vi "ramp.vi"(4 "DigNum Refnum":refnum<vi>, 5 "Bool Refnum Reset":refnum<vi>, 6 "Bool Refnum Start":refnum<vi>, 7 "Time Per Step":dbl[](array[numeric]), 8 "Pressures":dbl[](array[numeric])) -> ()   [LabVIEW 2018]
panel:
  out "Ramp Function 2":dbl(graph)
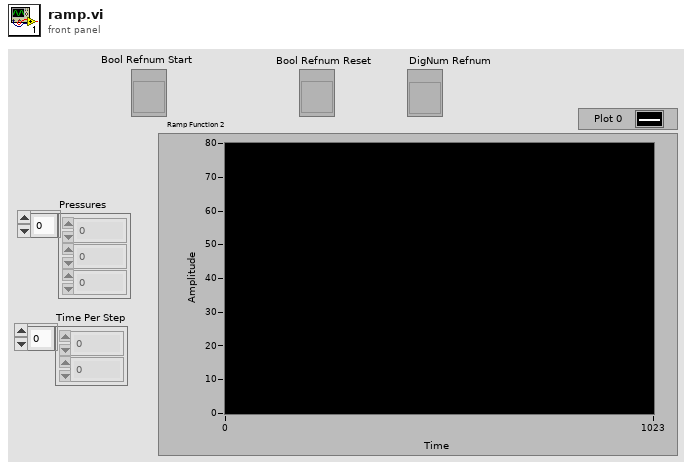
[diagram p1: front panel]
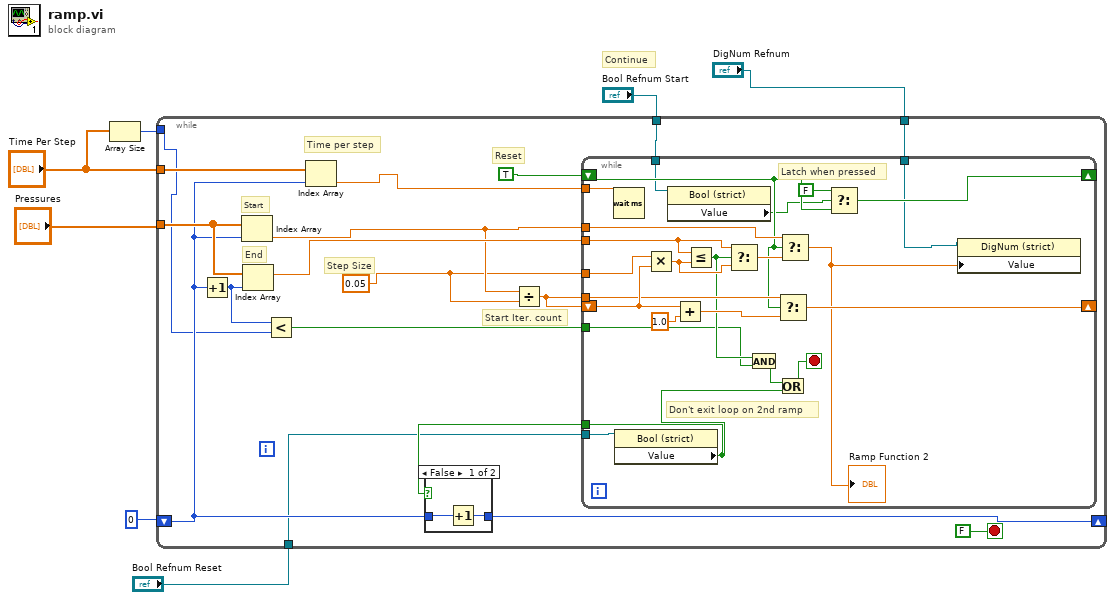
[diagram p0: block diagram]
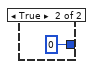
[diagram p2: hidden frame]
diagram:
  # "Continue"
  n1 = Array Size(array="Time Per Step") -> (size(s)=w5:i32)
  n2 = while {
    tunnel: "Pressures" -> [w25]
    tunnel: "Time Per Step" -> [w17]
    shift-right: [w12] -> _
    shift-left: 0 -> [w15]
    tunnel: w5 -> [w14]
    tunnel: "Bool Refnum Start" -> [w11]
    tunnel: "Bool Refnum Reset" -> [w8]
    tunnel: "DigNum Refnum" -> [w10]
    stop <- FALSE stop-if-true
    w22 = 0.05
    # "Reset"
    # "Time per step"
    # "Step Size"
    # "Start Iter. count"
    # "End"
    # "Start"
    n3 = Increment(x=w15) -> (x+1=w19:i32)
    n4 = Index Array(array=w25, index=w15) -> (element=w23:dbl)
    n5 = Index Array(array=w25, index=w19) -> (element=w24:dbl)
    n6 = Less?(x=w19, y=w14) -> (x < y?=w18:bool)
    n7 = Index Array(array=w17, index=w15) -> (element=w16:dbl)
    n8 = Divide(x=w23, y=w22) -> (x/y=w21:dbl)
    n9 = while {
      tunnel: w16 -> [w49]
      tunnel: w23 -> [w46]
      tunnel: w24 -> [w48]
      tunnel: w22 -> [w45]
      shift-right: [w40] -> _
      shift-left: w21 -> [w44]
      tunnel: w21 -> [w39]
      shift-right: [w37] -> _
      shift-left: TRUE -> [w36]
      tunnel: w18 -> [w34]
      tunnel: w11 -> [w31]
      tunnel: w10 -> [w29]
      tunnel: [w27] -> w9
      tunnel: w8 -> [w26]
      stop <- w32 stop-if-true
      # "Latch when pressed"
      # "Don't exit loop on 2nd ramp"
      n10 = Wait (ms)(milliseconds to wait=w49) -> ()  [unwired: 1 out]
      n11 = property class="Bool (strict)"(reference=w26) -> ("Value"=w27:bool)  [unwired: 1 in, 2 out]
      n12 = Multiply(x=w45, y=w44) -> (x*y=w47:dbl)
      n13 = property class="Bool (strict)"(reference=w31) -> ("Value"=w30:bool)  [unwired: 1 in, 2 out]
      n14 = Add(x=w44, y=1.0) -> (x+y=w41:dbl)
      n15 = Less Or Equal?(x=w48, y=w47) -> (x <= y?=w35:bool)
      n16 = Select(t=w48, s=w35, f=w47) -> (s? t:f=w42:dbl)
      n17 = And(x=w35, y=w34) -> (x .and. y?=w33:bool)
      n18 = Select(t=w39, s=w36, f=w41) -> (s? t:f=w40:dbl)
      n19 = Or(x=w33, y=w27) -> (x .or. y?=w32:bool)
      n20 = Select(t=w46, s=w36, f=w42) -> (s? t:f=w28:dbl)
      "Ramp Function 2" <- w28
      n21 = Select(t=FALSE, s=w30, f=w36) -> (s? t:f=w37:bool)
      n22 = property class="DigNum (strict)"(reference=w29, "Value"=w28) -> ()  [unwired: 1 in, 2 out]
    }
    n23 = case shown="False" w9 {
      tunnel: w15 -> [w51 _]
      tunnel: [w50 0] -> w12
      frame False {
        n24 = Increment(x=w51) -> (x+1=w50:i32)
      }
      frame True {
      }
    }
  }
